vi "HT3_Create.vi"(1 "Laser":i32[][](array[numeric]), 4 "Image Header in":T3, 5 "Save pt3":bool=TRUE, 6 "Measurement Type":T2(ring)=enum."Point Measurement", 7 "overwrite existing":bool, 8 "error in":errorcluster, 9 "Comment":string, 10 "ht3 Header in":T4={"Comment"="", "Binning"=0, "Offset"=0, "AcquisitionTime (ms)"=0, "HardwareSerial"=0, "SyncDivider"=0, "Resolution (ps)"=0.0, "CFD Settings"={"Sync Level"=150, "Sync ZeroX"=10, "Sync Offset"=-1000, "Chan Settings"=[{"CHx Level"=50, "CHx ZeroX"=10, "CHx Offset"=0}, {"CHx Level"=50, "CHx ZeroX"=10, "CHx Offset"=0}, {"CHx Level"=50, "CHx ZeroX"=10, "CHx Offset"=0}, {"CHx Level"=50, "CHx ZeroX"=10, "CHx Offset"=0}]}, "ModuleInfo"=[], "BaseResolution (ps)"=0.0, "RefClockSource"=0, "ChanInfo"=[], "SyncRate"=0, "InputsEnabled"=0}, 11 "File Path":path) -> (0 "error out":errorcluster, 2 "FileHeaderPos":T1, 3 "refnum out":refnum<file>)   [LabVIEW 2011]
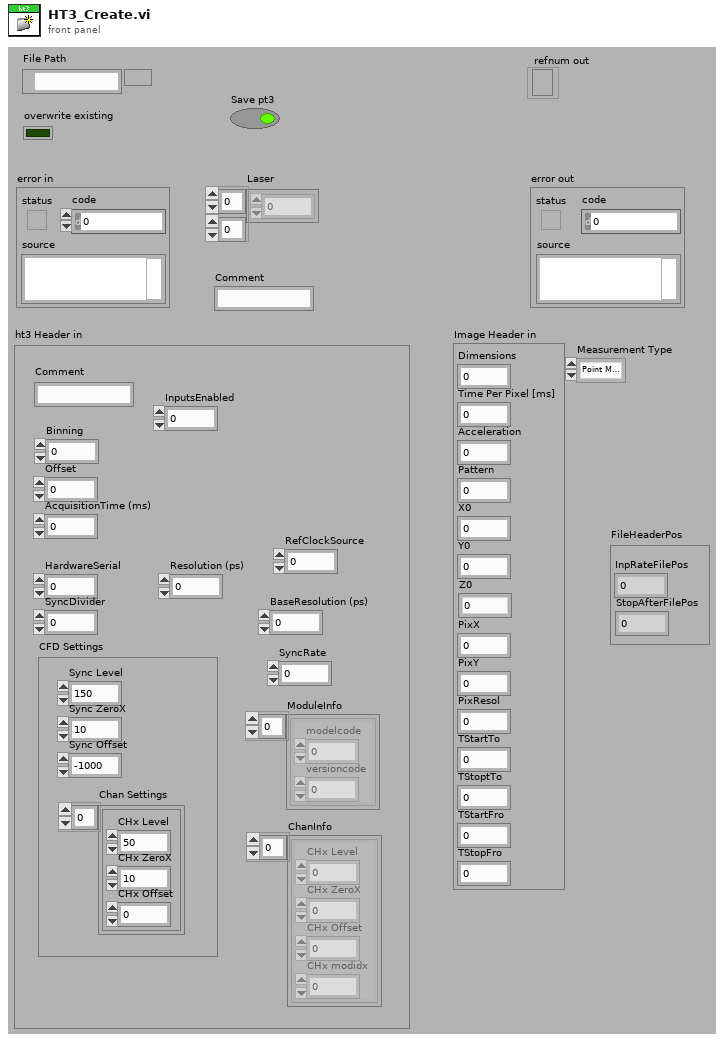
[diagram p1: front panel]
types:
  T1 = cluster{"InpRateFilePos":i64, "StopAfterFilePos":i64}
  T2 = enum16{"not a pt3 File", "Image File", "Point Measurement", "Auto Point", "Line Scan"}
  T3 = cluster{"Dimensions":i32, "Time Per Pixel [ms]":dbl, "Acceleration":i32, "Pattern":i32, "X0":sgl, "Y0":sgl, "Z0":dbl, "PixX":i32, "PixY":i32, "PixResol":sgl, "TStartTo":sgl, "TStoptTo":sgl, "TStartFro":sgl, "TStopFro":sgl}
  T4 = cluster{"Comment":string, "Binning":i32, "Offset":i32, "AcquisitionTime (ms)":i32, "HardwareSerial":i32, "SyncDivider":i32, "Resolution (ps)":dbl, "CFD Settings":cluster{"Sync Level":i32, "Sync ZeroX":i32, "Sync Offset":i32, "Chan Settings":cluster{"CHx Level":i32, "CHx ZeroX":i32, "CHx Offset":i32}[]}, "ModuleInfo":cluster{"modelcode":i32, "versioncode":i32}[], "BaseResolution (ps)":dbl, "RefClockSource":i32, "ChanInfo":cluster{"CHx Level":i32, "CHx ZeroX":i32, "CHx Offset":i32, "CHx modidx":i32}[], "SyncRate":i32, "InputsEnabled":i64}
  T5 = enum16{"big-endian, network order", "native, host order", "little-endian"}
  T6 = enum16{"open", "replace", "create", "open or create", "replace or create", "replace or create with confirmation"}
  T7 = cluster{"index of element":i32, "Bits per Record":i32, "ActiveCurve":i32, "MeasurementMode (3 = T3)":i32, "f":i32, "Binning":i32, "Resolution (ps)":dbl, "Offset":i32, "AcquisitionTime (ms)":i32, "StopAt":u32, "StopOnOvfl":i32, "Restart":i32, "DisplayLinLog":i32, "DisplayTimeAxisFrom":i32, "DisplayTimeAxisTo":i32, "DisplayCountAxisFrom":i32, "DisplayCountAxisTo":i32}
  T8 = cluster{"Sync Level":i32, "Sync ZeroX":i32, "Sync Offset":i32, "Chan Settings":cluster{"CHx Level":i32, "CHx ZeroX":i32, "CHx Offset":i32}[]}
  T9 = cluster{"CHx Level":i32, "CHx ZeroX":i32, "CHx Offset":i32, "CHx modidx":i32}[]
  T10 = cluster{"BaseResolution (ps)":dbl, "InputsEnabled":i64, i32, "RefClockSource":i32, "ExtDevices":i32, "MarkerSettings":i32, "SyncDivider":i32, "Sync Level":i32, "Sync ZeroX":i32, "Sync Offset":i32}
  T11 = cluster{"SyncRate":i32, "StopAfter":i32, "StopReason":i32, "f":i32, "NumRecords":i64}
  T12 = cluster{"offset (in bytes)":i64, "offset (in bytes)":i64}
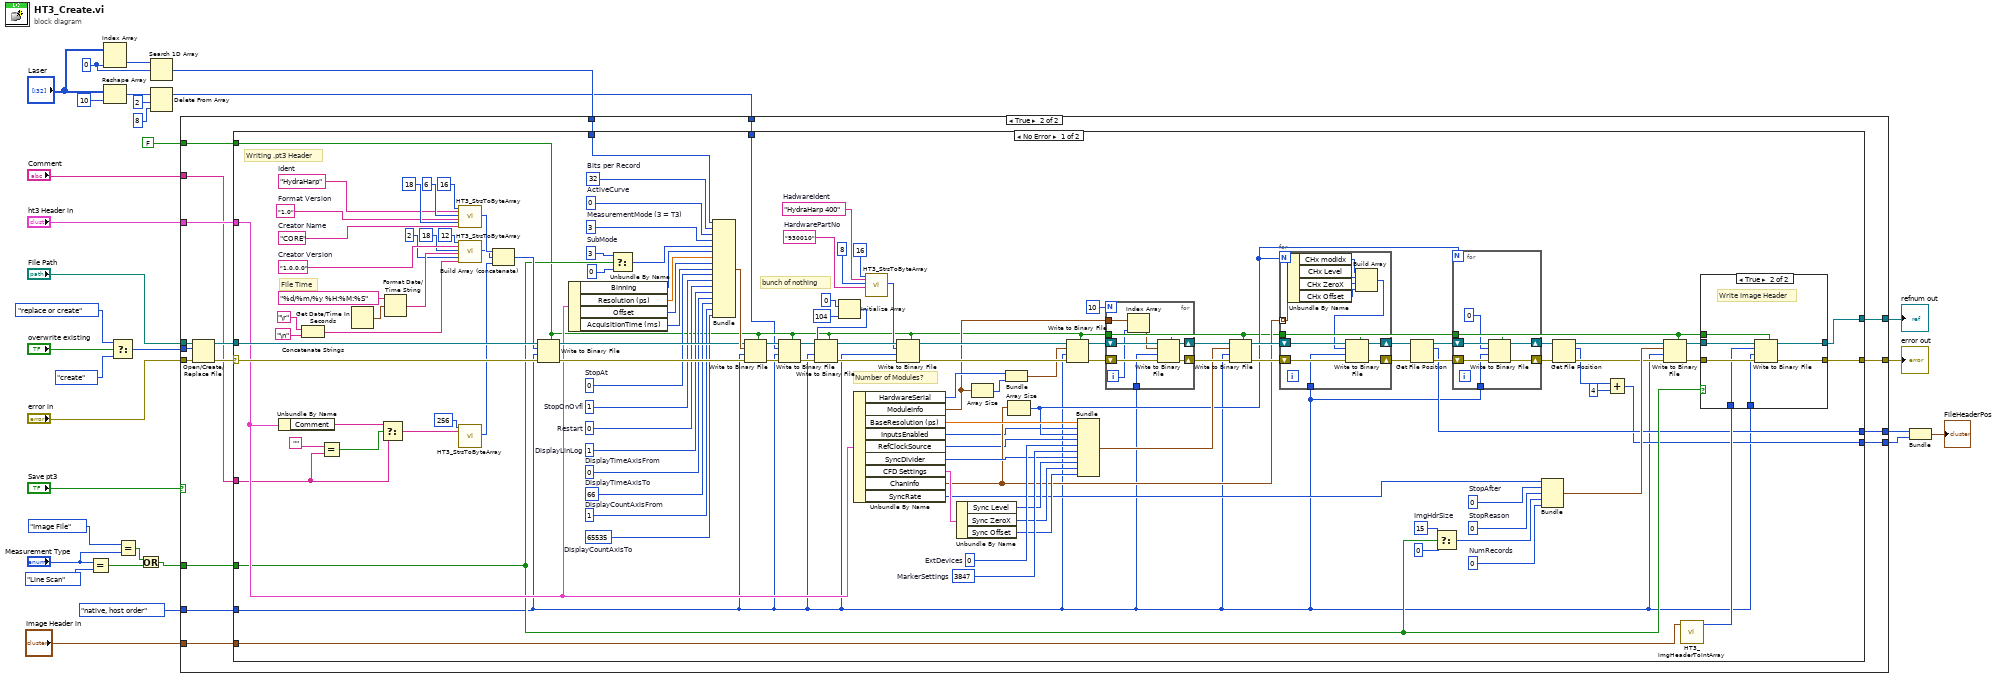
[diagram p0: block diagram]
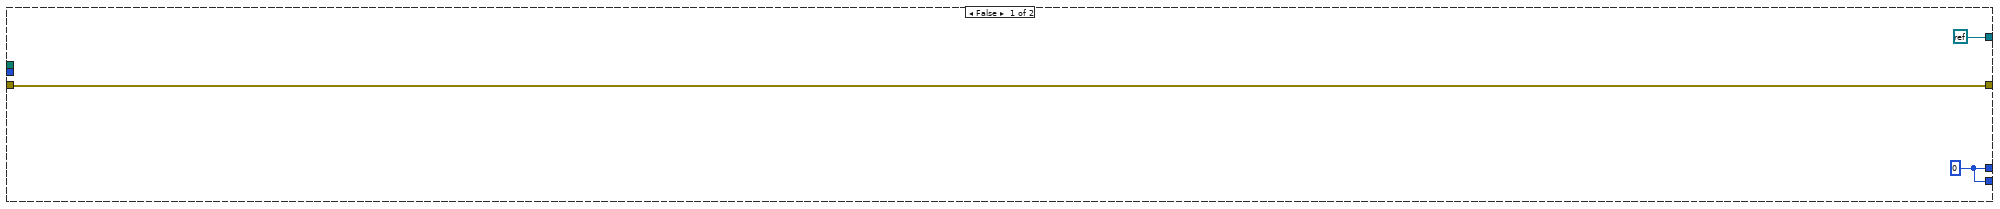
[diagram p2: hidden frame]
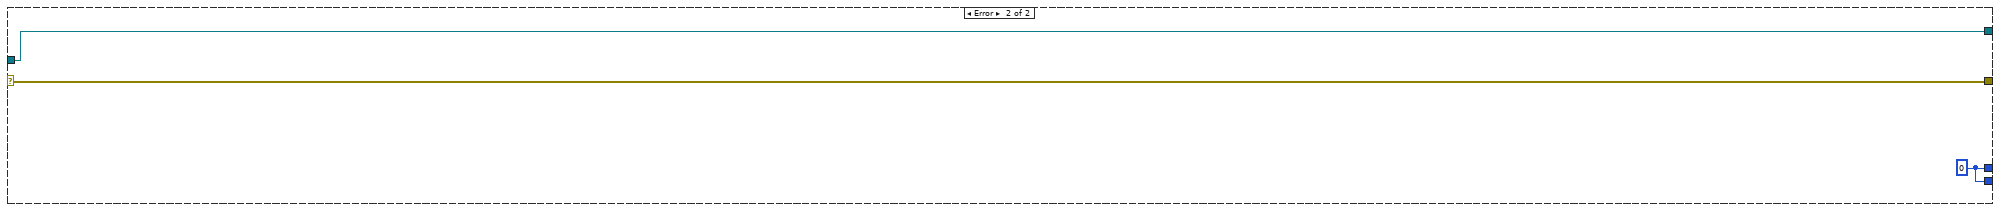
[diagram p4: hidden frame]
diagram:
  w5 = 0
  n1 = Equal?(x="Measurement Type", y=T2."Line Scan") -> (x = y?=w12:bool)
  n2 = Index Array(array="Laser", index (col)=w5) -> (element=w9:i32[])  [unwired: 1 in]
  n3 = Reshape Array("Laser", 10) -> (w6:i32[])
  n4 = Select(t=T6."replace or create" ("operation (0:open)"), s="overwrite existing", f=T6."create" ("operation (0:open)")) -> (s? t:f=w28:T6)
  n5 = Equal?(x=T2."Image File" ("y"), y="Measurement Type") -> (x = y?=w11:bool)
  n6 = Or(x=w11, y=w12) -> (x .or. y?=w10:bool)
  n7 = Search 1D Array(1D array=w9, element=w5) -> (index of element=w8:i32)  [unwired: 1 in]
  n8 = Delete From Array(array=w6, length=2, index=8) -> (array with subset deleted=w3:i32[])  [unwired: 1 out]
  n9 = case shown="True" "Save pt3" {
    tunnel: "File Path" -> [_ w52]
    tunnel: w28 -> [_ w51]
    tunnel: "error in" -> [w35 w50]
    tunnel: [w35 w48] -> w26
    tunnel: [refnum<k0> refnum w46] -> w25
    tunnel: "ht3 Header in" -> [_ w45]
    tunnel: T5."native, host order" ("byte order (0:big-endian, network order)") -> [_ w44]
    tunnel: FALSE ("prepend array or string size? (T)") -> [_ w43]
    tunnel: "Comment" -> [_ w42]
    tunnel: w10 -> [_ w41]
    tunnel: "Image Header in" -> [_ w40]
    tunnel: [w33 w39] -> w18
    tunnel: [w33 w38] -> w17
    tunnel: w8 -> [_ w37]
    tunnel: w3 -> [_ w36]
    frame False {
      w33 = i64 0 ("offset (in bytes)")
    }
    frame True {
      n10 = Open/Create/Replace File(file path (use dialog)=w52, error in=w50, operation (0:open)=w51) -> (refnum out=w47:refnum<file>, error out=w49:errorcluster)  [unwired: 4 out]
      n11 = case shown="No Error" w49 {
        selector: w49 -> [w173 w213]
        tunnel: [w106 w213] -> w48
        tunnel: w47 -> [w172 w212]
        tunnel: [w104 w212] -> w46
        tunnel: w45 -> [w120 _]
        tunnel: w44 -> [w54 _]
        tunnel: w43 -> [w55 _]
        tunnel: w42 -> [w64 _]
        tunnel: w41 -> [w108 _]
        tunnel: w40 -> [w109 _]
        tunnel: [w68 w211] -> w39
        tunnel: [w67 w211] -> w38
        tunnel: w37 -> [w59 _]
        tunnel: w36 -> [w53 _]
        frame No Error {
          w91 = 3847  # MarkerSettings
          w92 = 0  # ExtDevices
          w111 = 15  # ImgHdrSize
          w60 = i64 0  # NumRecords
          w118 = 0  # StopReason
          w119 = 0  # StopAfter
          w126 = "930010"  # HardwarePartNo
          w128 = "HydraHarp 400"  # HadwareIdent
          w136 = 65535  # DisplayCountAxisTo
          w137 = 1  # DisplayCountAxisFrom
          w138 = 66  # DisplayTimeAxisTo
          w139 = 0  # DisplayTimeAxisFrom
          w140 = 1  # DisplayLinLog
          w141 = 0  # Restart
          w142 = 1  # StopOnOvfl
          w143 = u32 0  # StopAt
          w113 = 3  # SubMode
          w147 = 3  # MeasurementMode (3 = T3)
          w148 = 0  # ActiveCurve
          w102 = 32  # Bits per Record
          w162 = "1.0.0.0"  # Creator Version
          w65 = "CORE"  # Creator Name
          w163 = "1.0"  # Format Version
          w164 = "HydraHarp"  # Ident
          # "Number of Modules?"
          # "bunch of nothing"
          # "File Time"
          # "Writing .pt3 Header"
          n12 = Unbundle By Name(w120) -> ("Comment"=w115:string)
          n13 = Concatenate Strings("\r", "\n") -> (w160:string)
          n14 = Equal?(x="", y=w64) -> (x = y?=w116:bool)
          n15 = Get Date/Time In Seconds() -> (seconds since 1Jan1904=w169:timestamp)
          n16 = Select(t=w115, s=w116, f=w64) -> (s? t:f=w114:string)
          n17 = Format Date/Time String(time format string (%c)="%d/%m/%y %H:%M:%S", seconds (now)=w169) -> (date/time string=w161:string)  [unwired: 1 out]
          n18 = call "HT3_StrsToByteArray.vi"("Length"=16, "String"=w164, "Length 2"=6 ("Length"), "String 2"=w163, "Length 3"=18 ("Length"), "String 3"=w65) -> ("Byte Array"=w156:u8[])  [unwired: 1 in, 12 out]
          n19 = call "HT3_StrsToByteArray.vi"("Length"=12, "String"=w162, "Length 2"=18 ("Length"), "String 2"=w161, "Length 3"=2 ("Length"), "String 3"=w160) -> ("Byte Array"=w155:u8[])  [unwired: 1 in, 12 out]
          n20 = call "HT3_StrsToByteArray.vi"("Length"=256, "String"=w114) -> ("Byte Array"=w153:u8[])  [unwired: 5 in, 12 out]
          n21 = Build Array (concatenate)(w156, w155, w153) -> (w152:u8[])
          n22 = Write to Binary File(file (use dialog)=w172, data=w152, error in=w173, 5:w55, 9:w54) -> (refnum out=w149:refnum<file>, error out=w150:errorcluster)  [unwired: 2 out]
          n23 = Unbundle By Name(w120) -> ("Binning"=w100:i32, "Resolution (ps)"=w146:dbl, "Offset"=w145:i32, "AcquisitionTime (ms)"=w144:i32)
          n24 = Select(t=w113, s=w108, f=0) -> (s? t:f=w101:i32)
          n25 = Bundle("index of element"=w59, "Bits per Record"=w102, "ActiveCurve"=w148, "MeasurementMode (3 = T3)"=w147, "f"=w101, "Binning"=w100, "Resolution (ps)"=w146, "Offset"=w145, "AcquisitionTime (ms)"=w144, "StopAt"=w143, "StopOnOvfl"=w142, "Restart"=w141, "DisplayLinLog"=w140, "DisplayTimeAxisFrom"=w139, "DisplayTimeAxisTo"=w138, "DisplayCountAxisFrom"=w137, "DisplayCountAxisTo"=w136) -> (w151:T7)  [unwired: 1 in]
          n26 = Write to Binary File(file (use dialog)=w149, data=w151, error in=w150, 5:w55, 9:w54) -> (refnum out=w57:refnum<file>, error out=w135:errorcluster)  [unwired: 2 out]
          n27 = Write to Binary File(file (use dialog)=w57, data=w53, error in=w135, 5:w55, 9:w54) -> (refnum out=w56:refnum<file>, error out=w58:errorcluster)  [unwired: 1 in, 1 out]
          n28 = Initialize Array(u8 0 ("element"), 104 ("dimension size")) -> (w132:u8[])
          n29 = Write to Binary File(file (use dialog)=w56, data=w132, error in=w58, 5:w55, 9:w54) -> (refnum out=w130:refnum<file>, error out=w131:errorcluster)  [unwired: 2 out]
          n30 = Unbundle By Name(w120) -> ("HardwareSerial"=w122:i32, "ModuleInfo"=w94:cluster{"modelcode":i32, "versioncode":i32}[], "BaseResolution (ps)"=w93:dbl, "InputsEnabled"=w61:i64, "RefClockSource"=w62:i32, "SyncDivider"=w90:i32, "CFD Settings"=w89:T8, "ChanInfo"=w82:T9, "SyncRate"=w81:i32)
          n31 = call "HT3_StrsToByteArray.vi"("Length"=16, "String"=w128, "Length 2"=8, "String 2"=w126) -> ("Byte Array"=w129:u8[])  [unwired: 3 in, 12 out]
          n32 = Write to Binary File(file (use dialog)=w130, data=w129, error in=w131, 5:w55, 9:w54) -> (refnum out=w123:refnum<file>, error out=w124:errorcluster)  [unwired: 2 out]
          n33 = Unbundle By Name(w89) -> ("Sync Level"=w88:i32, "Sync ZeroX"=w87:i32, "Sync Offset"=w86:i32)
          n34 = Array Size(array=w94) -> (size(s)=w95:i32)
          n35 = Bundle("HardwareSerial"=w122, w95) -> (w121:cluster{"HardwareSerial":i32, i32})  [unwired: 1 out]
          n36 = Array Size(array=w82) -> (size(s)=w79:i32)
          n37 = Write to Binary File(file (use dialog)=w123, data=w121, error in=w124, 5:w55, 9:w54) -> (refnum out=w99:refnum<file>, error out=w98:errorcluster)  [unwired: 2 out]
          n38 = Bundle("BaseResolution (ps)"=w93, "InputsEnabled"=w61, w79, "RefClockSource"=w62, "ExtDevices"=w92, "MarkerSettings"=w91, "SyncDivider"=w90, "Sync Level"=w88, "Sync ZeroX"=w87, "Sync Offset"=w86) -> (w85:T10)  [unwired: 1 in]
          n39 = for {
            N: 10 -> [_]
            tunnel: w55 -> [w197]
            shift-right: [w198] -> w96
            shift-left: w99 -> [w201]
            shift-right: [w199] -> w97
            shift-left: w98 -> [w200]
            tunnel: w94 -> [w195]
            tunnel: w54 -> [w196]
            i -> [w194]
            n40 = Index Array(array=w195, index=w194) -> (element=w193:cluster{"modelcode":i32, "versioncode":i32})
            n41 = Write to Binary File(file (use dialog)=w201, data=w193, error in=w200, 5:w197, 9:w196) -> (refnum out=w198:refnum<file>, error out=w199:errorcluster)  [unwired: 2 out]
          }
          n42 = Write to Binary File(file (use dialog)=w96, data=w85, error in=w97, 5:w55, 9:w54) -> (refnum out=w84:refnum<file>, error out=w83:errorcluster)  [unwired: 2 out]
          n43 = for {
            N: w79 -> [_]
            tunnel: w55 -> [w188]
            shift-right: [w189] -> w78
            shift-left: w84 -> [w192]
            shift-right: [w190] -> w77
            shift-left: w83 -> [w191]
            tunnel: w82 -> [w186] mode=indexing
            tunnel: w54 -> [w187]
            n44 = Unbundle By Name(w186) -> ("CHx modidx"=w185:i32, "CHx Level"=w184:i32, "CHx ZeroX"=w183:i32, "CHx Offset"=w182:i32)
            n45 = Build Array(w185, w184, w183, w182) -> (w181:i32[])
            n46 = Write to Binary File(file (use dialog)=w192, data=w181, error in=w191, 5:w188, 9:w187) -> (refnum out=w189:refnum<file>, error out=w190:errorcluster)  [unwired: 2 out]
          }
          n47 = Get File Position(4:w77, 7:w78) -> (0:w76:errorcluster, 2:w68:i64, 3:w75:refnum<file>)
          n48 = Select(t=w111, s=w108, f=0) -> (s? t:f=w80:i32)
          n49 = for {
            N: w79 -> [_]
            tunnel: w55 -> [w176]
            shift-right: [w177] -> w73
            shift-left: w75 -> [w180]
            shift-right: [w178] -> w74
            shift-left: w76 -> [w179]
            tunnel: w54 -> [w175]
            n50 = Write to Binary File(file (use dialog)=w180, data=0, error in=w179, 5:w176, 9:w175) -> (refnum out=w177:refnum<file>, error out=w178:errorcluster)  [unwired: 2 out]
          }
          n51 = Bundle("SyncRate"=w81, "StopAfter"=w119, "StopReason"=w118, "f"=w80, "NumRecords"=w60) -> (w117:T11)  [unwired: 1 in]
          n52 = Get File Position(4:w74, 7:w73) -> (0:w71:errorcluster, 2:w70:i64, 3:w72:refnum<file>)
          n53 = Add(x=w70, y=i64 4) -> (x+y=w67:i64)
          n54 = Write to Binary File(file (use dialog)=w72, data=w117, error in=w71, 5:w55, 9:w54) -> (refnum out=w105:refnum<file>, error out=w107:errorcluster)  [unwired: 2 out]
          n55 = call "HT3_ImgHeaderToIntArray.vi"("Image Header"=w109) -> ("Array"=w103:i32[])  [unwired: 10 out]
          n56 = case shown="True" w108 {
            tunnel: w107 -> [w202 w210]
            tunnel: [w202 w209] -> w106
            tunnel: w105 -> [w203 w208]
            tunnel: [w203 w207] -> w104
            tunnel: w55 -> [_ w206]
            tunnel: w103 -> [_ w205]
            tunnel: w54 -> [_ w204]
            frame False {
            }
            frame True {
              # "Write Image Header"
              n57 = Write to Binary File(file (use dialog)=w208, data=w205, error in=w210, 5:w206, 9:w204) -> (refnum out=w207:refnum<file>, error out=w209:errorcluster)  [unwired: 2 out]
            }
          }
        }
        frame Error {
          w211 = i64 0 ("offset (in bytes)")
        }
      }
    }
  }
  "refnum out" <- w25
  "error out" <- w26
  n58 = Bundle("offset (in bytes)"=w18, "offset (in bytes)"=w17) -> (→"FileHeaderPos":T12)  [unwired: 1 in]
